vi "UMB_CluterToArrays.vi"(11 "data array [mag, phase (deg)]":cluster{"magnitude":dbl, "phase":dbl}[](array[cluster])) -> (2 "Phase":dbl[](array[numeric]), 3 "Magnitude":dbl[](array[numeric]))   [LabVIEW 2012]
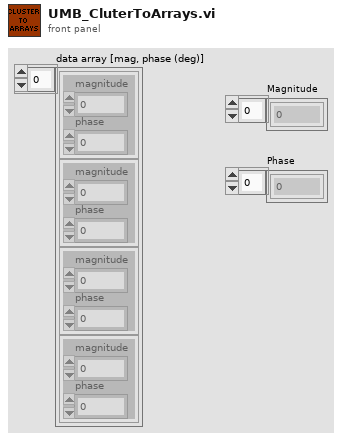
[diagram p1: front panel]
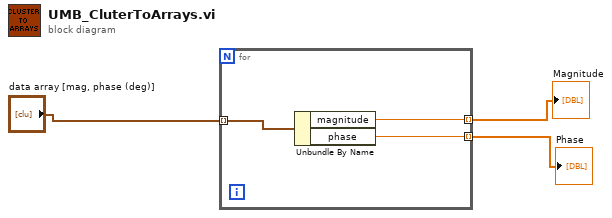
[diagram p0: block diagram]
diagram:
  n1 = for {
    tunnel: "data array [mag, phase (deg)]" -> [w6] mode=indexing
    tunnel: [w5] -> w2 mode=indexing
    tunnel: [w4] -> w1 mode=indexing
    n2 = Unbundle By Name(w6) -> ("magnitude"=w5:dbl, "phase"=w4:dbl)
  }
  "Magnitude" <- w2
  "Phase" <- w1
